vi "Calc resulting acq length.vi"(8 "error in (no error)":errorcluster, 11 "XYZ_Coordinates":T1[](array[typedef]) {"ROI group ID" format="%#_6f"; "Laser Power (%)" format="%#_6f"; "Zoom" format="%#_6f"; "Frame Size" format="%#_6f"; "Number of lines" format="%#_6f"; "Composite ID" format="%#_6f"; "Angle (deg)" format="%#_6f"; "ROI Time (ns)" format="%#_6f"; "ROI ID" format="%#_6f"; "Pixels in ROI" format="%#_6f"; "ROI index" format="%#_6f"; "Z stop" format="%#_6f"; "Y stop" format="%#_6f"; "X stop" format="%#_6f"; "Z start" format="%#_6f"; "X start" format="%#_6f"; "Y start" format="%#_6f"}) -> (0 "error out":errorcluster, 3 "Output cluster":T2={"Imaging Protocol"=enum."AOL Z-Stack", "Number of POI"=0, "Number of Miniscans"=0, "Number of Trials"=0, "Number of Cycles "=0, "# Averaged Frames"=0, "Laser power (%)"=0, "Pockels"=0.0, "Acquisition Length (sec)"=0.0, "Fill time (us)"=0.0, "POI Dwell time (us)"=0.0, "Miniscan Dwell time per pixel (us)"=0.0, "PMT 1"=0.0, "PMT 2"=0.0, "Back Apperture"=0.0, "Frame Size"=0, "Center Frequency"=0.0, "Field of View"=0.0, "DwellTime (us)"=0.0, "Wavelength (nm)"=0.0, "Zoom"=0.0, "AOL Z"=0.0, "AOL Mode"=enum."Raster", "GridXY"=0.0, "GridZ"=0.0, "TriggerPeriod (sec)"=0.0, "Number of Pixels in Miniscan"=0, "Experiment folder path"=path "", "X centre"=0.0, "Y centre"=0.0, "Angle (degrees)"=0.0, "Plane Mode"=0, "Threshold"=[], "Regenerate Chirps"=FALSE, "Rectangle ROI length (pixels)"=0, "Rectangle ROI height (pixels)"=0, "AOD fill"=0, "Samples Wait after Trigger"=0, "StartUp Delay"=0, "Slip Cycle"=163840, "Add Cycle"=FALSE} {"Plane Mode" items=["XY Plane"]; "Frame Size" items=["100X100"=100, "128X128"=128, "200X200"=200, "256X256"=256, "512X512"=512, "1024x1024"=1024, "2048x2048"=2048]; "Back Apperture" format="%#.6g"; "Pockels" format="%#.6g"; "PMT 2" format="%#.6g"; "PMT 1" format="%#.6g"; "Angle (degrees)" format="%#.6g"; "POI Dwell time (us)" format="%#.6g"})   [LabVIEW 2013]
uses:
  Typedefs/Controls/AOL_Globals.ctl
  Typedefs/Imaging Protocols enum.ctl
  Typedefs/Frame Size.ctl
  Typedefs/AOL modes.ctl
  Typedefs/Plane Mode.ctl
  Visualisation/Functional Imaging Viewer/Typedefs/ROI parameters data type.ctl
  Global Variables/General Globals.vi
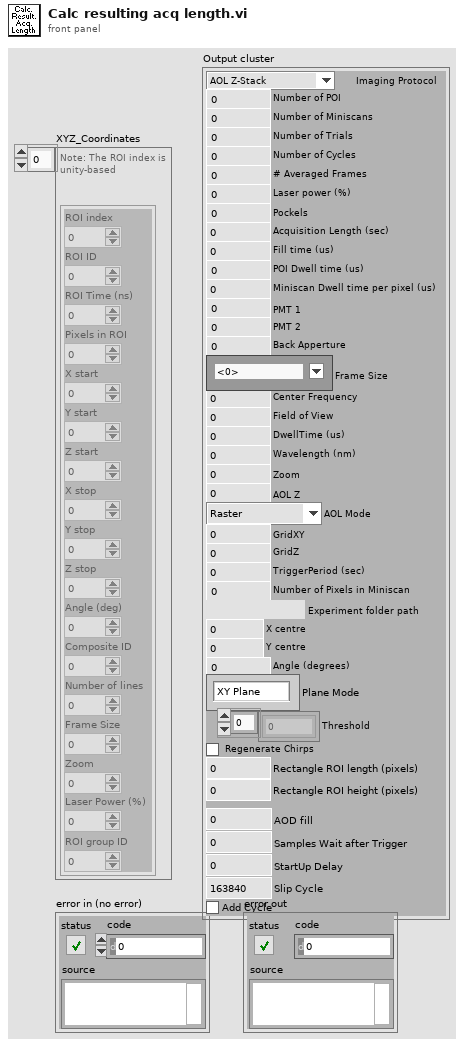
[diagram p1: front panel]
types:
  T1 = typedef "ROI parameters data type.ctl" = cluster{"ROI index":dbl, "ROI ID":dbl, "ROI Time (ns)":dbl, "Pixels in ROI":dbl, "X start":dbl, "Y start":dbl, "Z start":dbl, "X stop":dbl, "Y stop":dbl, "Z stop":dbl, "Angle (deg)":dbl, "Composite ID":dbl, "Number of lines":dbl, "Frame Size":dbl, "Zoom":dbl, "Laser Power (%)":dbl, "ROI group ID":dbl}
  T2 = typedef "AOL_Globals.ctl" = cluster{"Imaging Protocol":T3, "Number of POI":u16, "Number of Miniscans":u16, "Number of Trials":u16, "Number of Cycles ":u64, "# Averaged Frames":u16, "Laser power (%)":u8, "Pockels":dbl, "Acquisition Length (sec)":dbl, "Fill time (us)":dbl, "POI Dwell time (us)":dbl, "Miniscan Dwell time per pixel (us)":dbl, "PMT 1":dbl, "PMT 2":dbl, "Back Apperture":dbl, "Frame Size":T4, "Center Frequency":dbl, "Field of View":dbl, "DwellTime (us)":dbl, "Wavelength (nm)":dbl, "Zoom":dbl, "AOL Z":dbl, "AOL Mode":T5, "GridXY":dbl, "GridZ":dbl, "TriggerPeriod (sec)":dbl, "Number of Pixels in Miniscan":u16, "Experiment folder path":path, "X centre":dbl, "Y centre":dbl, "Angle (degrees)":dbl, "Plane Mode":T6, "Threshold":u16[], "Regenerate Chirps":bool, "Rectangle ROI length (pixels)":u16, "Rectangle ROI height (pixels)":u16, "AOD fill":u16, "Samples Wait after Trigger":u16, "StartUp Delay":i32, "Slip Cycle":u32, "Add Cycle":bool}
  T3 = typedef "Imaging Protocols enum.ctl" = enum16{"AOL Z-Stack", "Motor Z Stack", "Functional Acquisition", "Single Plane Acquisition", "Volume Acquisition", "Live Imaging", "Live Plane Imaging", "Live Volume Imaging"}
  T4 = typedef "Frame Size.ctl" = u16
  T5 = typedef "AOL modes.ctl" = enum16{"Raster", "Structural", "Pointing", "Mini Scan", "Alignment"}
  T6 = typedef "Plane Mode.ctl" = u16
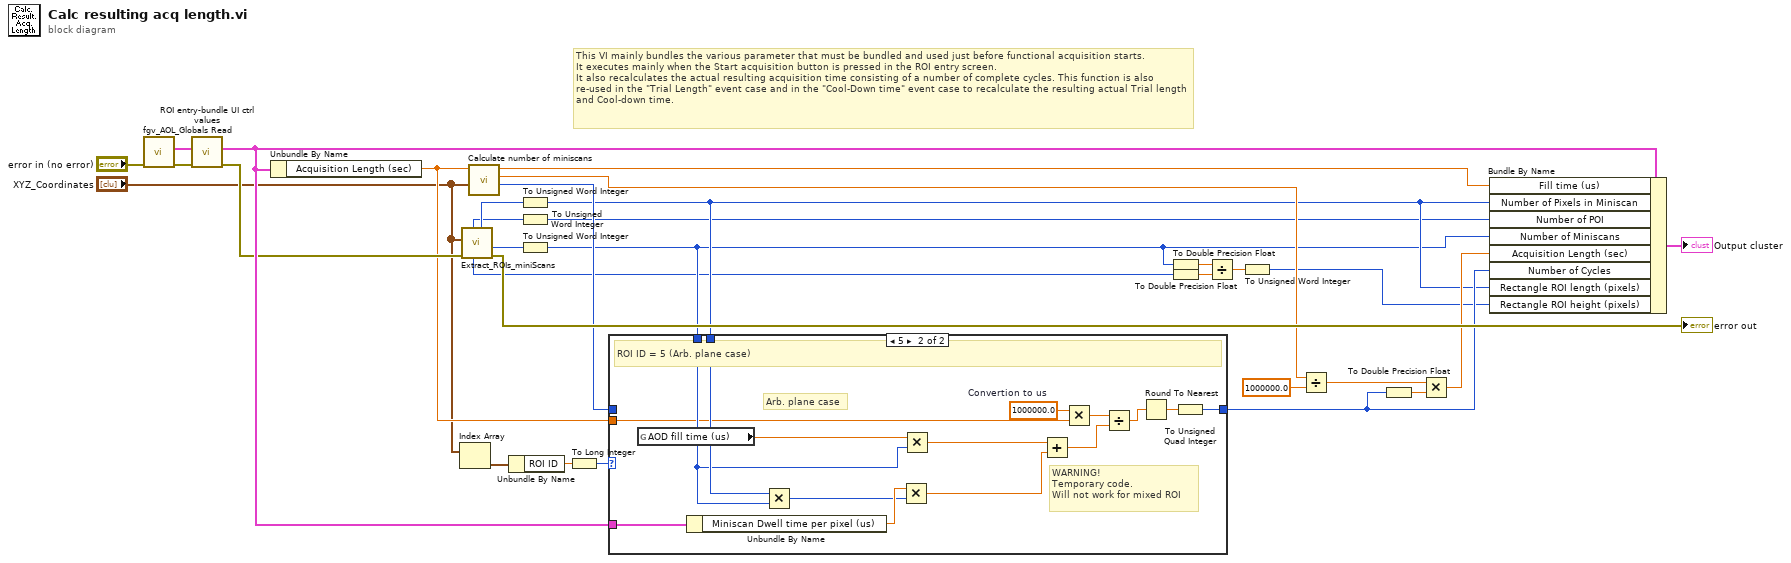
[diagram p0: block diagram]
diagram:
  # "This VI mainly bundles the various parameter that must be bundled and used just before functional acquisition starts.\nIt executes mainly when the Start acquisition button is pressed in the ROI entry screen.\nIt also recalculates the actual resulting acquisition time consisting of a number of complete cycles. This function is also re-used in the \"Trial Length\" event case and in the \"Cool-Down time\" event case to recalculate the resulting actual Trial length and Cool-down time."
  n1 = call "fgv_AOL_Globals Read.vi"("error in (no error)"="error in (no error)") -> ("error out"=w28:errorcluster, "AOL_Globals"=w29:T2)  [unwired: 8 in, 1 out]
  n2 = call "ROI entry-bundle UI ctrl values.vi"("error in (no error)"=w28, "Input cluster"=w29) -> ("Error Out"=w27:errorcluster, "Output cluster"=w31:T2)  [unwired: 8 in]
  n3 = Unbundle By Name(w31) -> ("Acquisition Length (sec)"=w26:dbl)
  n4 = Index Array(array="XYZ_Coordinates") -> (element=w17:T1)  [unwired: 1 in]
  n5 = call "Extract_ROIs_miniScans.vi"("error in (no error)"=w27, "ROI Attributes"="XYZ_Coordinates") -> ("error out"=→"error out":errorcluster, "Total number of miniscans"=w21:i32, "Number of pixels in single X miniscan"=w20:i32, "number of rectangles"=w5:i32, "number of POI"=w19:i32)  [unwired: 2 in, 3 out]
  n6 = call "Calculate number of miniscans.vi"("XYZ Coordinates"="XYZ_Coordinates", "Acquisition length (sec)"=w26) -> ("Number of cycles"=w18:u64, "Cycle time (us)"=w10:dbl, "AOD fill time (us)"=w22:dbl)  [unwired: 7 in]
  n7 = Unbundle By Name(w17) -> ("ROI ID"=w16:dbl)
  n8 = To Unsigned Word Integer(number=w20) -> (unsigned 16bit integer=w8:u16)
  n9 = To Unsigned Word Integer(number=w19) -> (unsigned 16bit integer=w6:u16)
  n10 = To Unsigned Word Integer(number=w21) -> (unsigned 16bit integer=w7:u16)
  n11 = To Long Integer(number=w16) -> (32bit integer=w15:i32)
  n12 = case shown="5" w15 {
    tunnel: w8 -> [_ w45]
    tunnel: w7 -> [_ w44]
    tunnel: w31 -> [_ w43]
    tunnel: w26 -> [_ w34]
    tunnel: [w32 w33] -> w11
    tunnel: w18 -> [w32 _]
    frame Default {
      # "ROI ID is not 5 (i.e. All other ROI types)"
    }
    frame 5 {
      w39 = 1000000.0  # Convertion to us
      # "WARNING!\nTemporary code.\nWill not work for mixed ROI"
      # "Arb. plane case"
      # "ROI ID = 5 (Arb. plane case)"
      n13 = global read "General Globals.vi" "AOD fill time (us)"() -> (w47:dbl)
      n14 = Unbundle By Name(w43) -> ("Miniscan Dwell time per pixel (us)"=w42:dbl)
      n15 = Multiply(x=w45, y=w44) -> (x*y=w41:u16)
      n16 = Multiply(x=w42, y=w41) -> (x*y=w40:dbl)
      n17 = Multiply(x=w47, y=w44) -> (x*y=w46:dbl)
      n18 = Add(x=w46, y=w40) -> (x+y=w35:dbl)
      n19 = Multiply(x=w39, y=w34) -> (x*y=w38:dbl)
      n20 = Divide(x=w38, y=w35) -> (x/y=w36:dbl)
      n21 = Round To Nearest(number=w36) -> (nearest integer value=w37:dbl)
      n22 = To Unsigned Quad Integer(1:w37) -> (0:w33:u64)
    }
  }
  n23 = To Double Precision Float(number=w7) -> (double precision float=w3:dbl)
  n24 = To Double Precision Float(number=w5) -> (double precision float=w2:dbl)
  n25 = Divide(x=w3, y=w2) -> (x/y=w4:dbl)
  n26 = To Unsigned Word Integer(number=w4) -> (unsigned 16bit integer=w1:u16)
  n27 = Divide(x=w10, y=1000000.0) -> (x/y=w12:dbl)
  n28 = To Double Precision Float(number=w11) -> (double precision float=w9:dbl)
  n29 = Multiply(x=w12, y=w9) -> (x*y=w14:dbl)
  n30 = Bundle By Name(cluster=w31, "Fill time (us)"=w22, "Number of Pixels in Miniscan"=w8, "Number of POI"=w6, "Number of Miniscans"=w7, "Acquisition Length (sec)"=w14, "Number of Cycles"=w11, "Rectangle ROI length (pixels)"=w8, "Rectangle ROI height (pixels)"=w1) -> (→"Output cluster":T2)
